vi "Launch Nested Actors.vi"(8 "error in (no error)":errorcluster, 11 "Interlock Chain in":refnum<class "Interlock Chain.lvclass">) -> (0 "error out":errorcluster, 3 "Interlock Chain out":refnum<class "Interlock Chain.lvclass">)   [LabVIEW 2015, in "Interlocks.lvlib" / "Interlock Chain.lvclass"]
uses:
  Interlock Chain.lvclass
  <vilib>/ActorFramework/Actor/Actor.lvclass/Actor.ctl
  <vilib>/ActorFramework/Message Enqueuer/Message Enqueuer.lvclass/Message Enqueuer.ctl
  Interlock Chain.lvclass/Interlock Chain.ctl
  Interlock Chain Messages/Launch Interlock Msg/Launch Interlock Msg.lvclass/Launch Interlock Msg.ctl
  <vilib>/ActorFramework/Message Enqueuer/Init from Existing Queue.vi
  <vilib>/ActorFramework/Message Enqueuer/Enqueue.vi
  <vilib>/ActorFramework/Message Priority Queue/Priority Enqueue.vi
  <vilib>/ActorFramework/Message Enqueuer/Message Enqueuer.lvclass
  Interlock Chain Messages/Launch Interlock Msg/Launch Interlock Msg.lvclass
  <vilib>/ActorFramework/Actor/Actor.lvclass
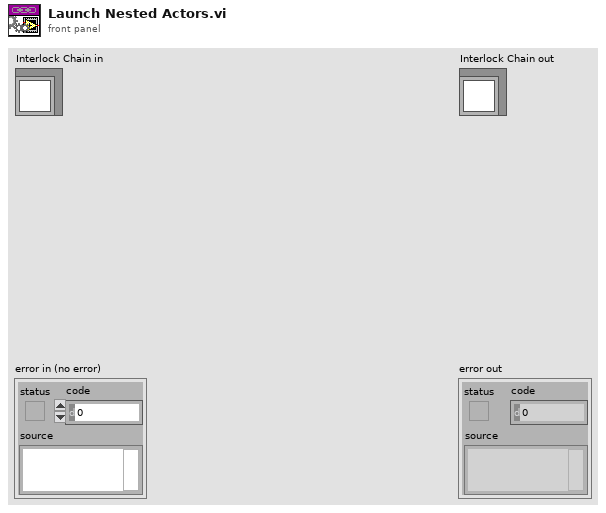
[diagram p1: front panel]
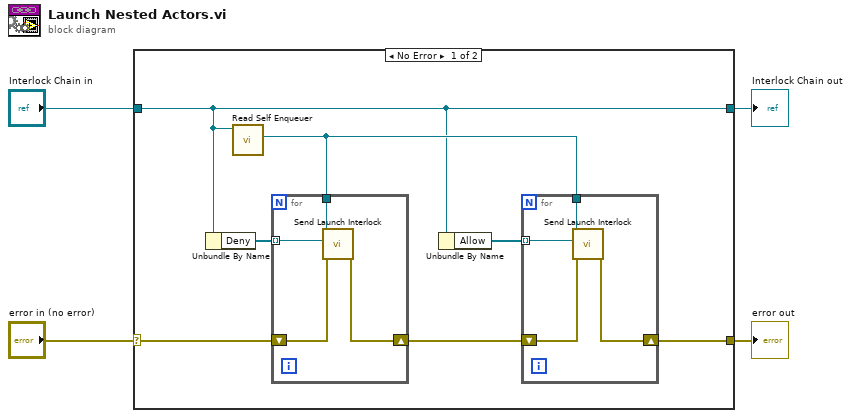
[diagram p0: block diagram]
diagram:
  n1 = case shown="No Error" "error in (no error)" {
    selector: "error in (no error)" -> [w10 w21]
    tunnel: [w5 w21] -> w3
    tunnel: [w6 w20] -> w1
    tunnel: "Interlock Chain in" -> [w6 w20]
    frame No Error {
      n2 = Unbundle By Name(w6) -> ("Deny"=w11:refnum<class "Interlock.lvclass">[])
      n3 = call <vilib>:"Read Self Enqueuer.vi"("Actor"=w6) -> ("Self Enqueuer"=w8:refnum<class "Message Enqueuer.lvclass">)  [unwired: 10 in]
      n4 = for {
        tunnel: w11 -> [w19] mode=indexing
        tunnel: w8 -> [w18]
        shift-right: [w16] -> w9
        shift-left: w10 -> [w17]
        n5 = call "Send Launch Interlock.vi"("error in (no error)"=w17, "Interlocks.lvlib:Interlock.lvclass"=w19, "Message Enqueuer"=w18) -> ("error out"=w16:errorcluster)  [unwired: 7 in, 1 out]
      }
      n6 = Unbundle By Name(w6) -> ("Allow"=w7:refnum<class "Interlock.lvclass">[])
      n7 = for {
        tunnel: w7 -> [w15] mode=indexing
        tunnel: w8 -> [w14]
        shift-right: [w12] -> w5
        shift-left: w9 -> [w13]
        n8 = call "Send Launch Interlock.vi"("error in (no error)"=w13, "Interlocks.lvlib:Interlock.lvclass"=w15, "Message Enqueuer"=w14) -> ("error out"=w12:errorcluster)  [unwired: 7 in, 1 out]
      }
    }
    frame Error {
    }
  }
  "error out" <- w3
  "Interlock Chain out" <- w1
